vi "aboutProgram (SubVI).vi"(10 "About_prg in":T1, 11 "Application Directory":path) -> (3 "About_prg out":T1)   [LabVIEW 2017]
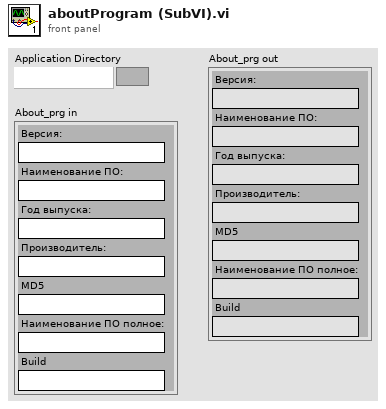
[diagram p1: front panel]
types:
  T1 = cluster{"Версия:":string, "Наименование ПО:":string, "Год выпуска:":string, "Производитель:":string, "MD5":string, "Наименование ПО полное:":string, "Build":string}
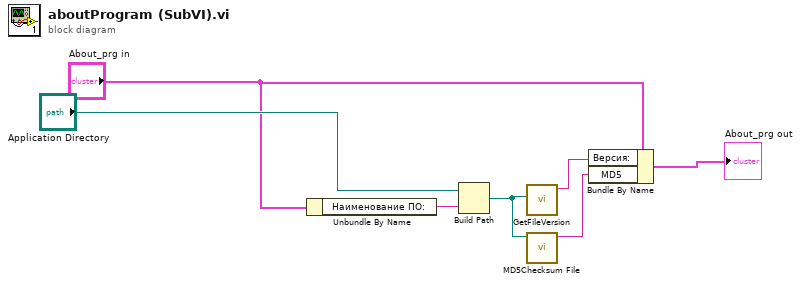
[diagram p0: block diagram]
diagram:
  n1 = Unbundle By Name("About_prg in") -> ("Наименование ПО:"=w3:string)
  n2 = Build Path(base path="Application Directory", name or relative path=w3) -> (appended path=w2:path)
  n3 = call "GetFileVersion.vi"("path"=w2) -> ("Full version"=w4:string)  [unwired: 10 in]
  n4 = call <vilib>:"MD5Checksum File.vi"("Path"=w2) -> ("MD5 message-digest"=w1:string)  [unwired: 9 in, 1 out]
  n5 = Bundle By Name(cluster="About_prg in", "Версия:"=w4, "MD5"=w1) -> (→"About_prg out":T1)
